vi "Set heartbeat table.vi"(4 "Heartbeat table":T1(array[cluster]) {"Period" format="%#.3g"}, 7 "CANopen in":refnum<class "CANopen.lvclass">) -> (3 "CANopen out":refnum<class "CANopen.lvclass">)   [LabVIEW 2023, in "canopen.lvlib" / "CANopen.lvclass"]
doc: "Sets the table where the heartbeat watchdog states are stored and updated."
uses:
  CANopen.lvclass
  CANopen.lvclass/CANopen.ctl
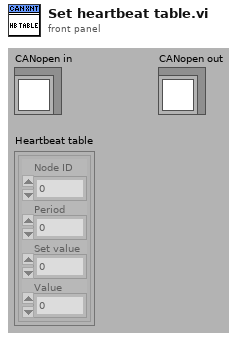
[diagram p1: front panel]
types:
  T1 = cluster{"Node ID":u8, "Period":dbl, "Set value":i16, "Value":i16}[]
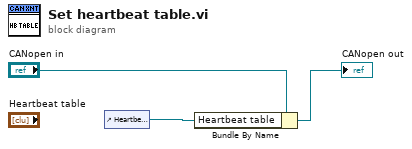
[diagram p0: block diagram]
diagram:
  n1 = control-ref of="Heartbeat table"() -> (w1:refnum<vi>)
  n2 = Bundle By Name(cluster="CANopen in", "Heartbeat table"=w1) -> (→"CANopen out":refnum<class "CANopen.lvclass">)
